vi "Insert.vi"(8 "error in (no error)":errorcluster, 9 "Item":refnum<class>, 10 "Index":i32, 11 "ListImp in":refnum<class "ListImp.lvclass">) -> (0 "error out":errorcluster, 3 "ListImp out":refnum<class "ListImp.lvclass">)   [LabVIEW 2013, in "LapDog.Collections.v1.Lists.lvlib" / "ListImp.lvclass"]
doc: "Inserts an item into the list at the location specified by Index, increasing the index of all items after the specified index by 1. If Index = -1 or Index = Count, the item is added to the end of the list. If Index < -1 or Index > Count, error 510201 is returned."
uses:
  ListImp.lvclass
  ListImp.lvclass/ListImp.ctl
  LapDog.Collections.Common/LapDog.Collections.v1.Common.lvlib
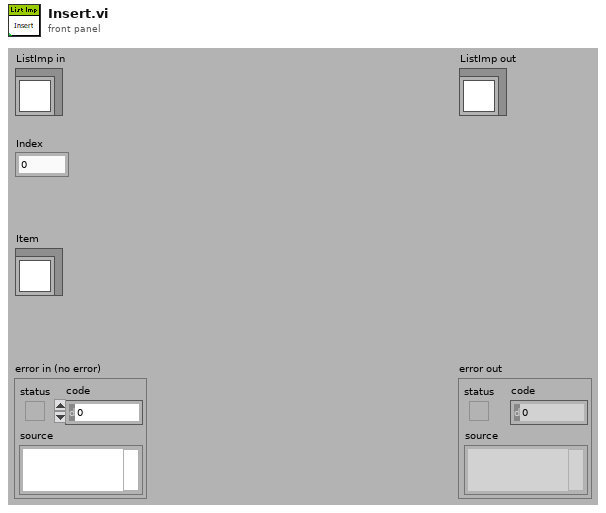
[diagram p1: front panel]
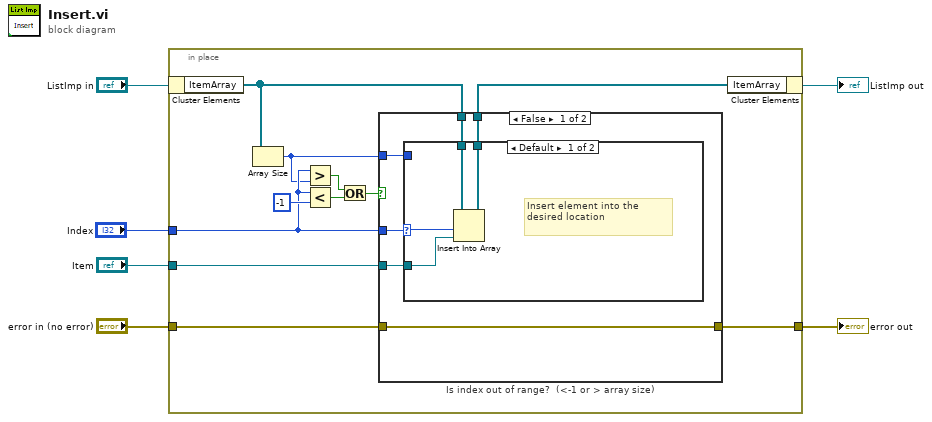
[diagram p0: block diagram]
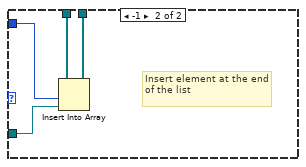
[diagram p2: hidden frame]
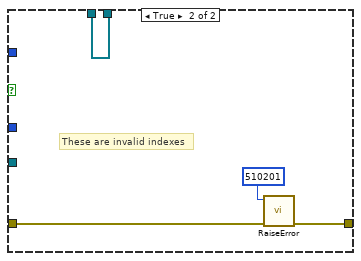
[diagram p3: hidden frame]
diagram:
  n1 = in-place {
    in-place-border: "Item" -> [w8]
    in-place-border: "Index" -> [w11]
    in-place-border: "error in (no error)" -> [w13]
    in-place-border: [w12] -> w3
    n2 = in-place-cluster #1("ListImp in") -> ("ItemArray"=w10:refnum<class>[])
    n3 = Array Size(array=w10) -> (size(s)=w7:i32)
    n4 = Greater?(x=w11, y=w7) -> (0:w15:bool)
    n5 = Less?(x=w11, y=-1) -> (x < y?=w16:bool)
    n6 = Or(x=w15, y=w16) -> (x .or. y?=w14:bool)
    n7 = case "Is index out of range?  (<-1 or > array size)" shown="False" w14 {
      tunnel: w13 -> [w23 w34]
      tunnel: [w23 w33] -> w12
      tunnel: w11 -> [w22 _]
      tunnel: w10 -> [w21 w32]
      tunnel: [w20 w32] -> w9
      tunnel: w8 -> [w19 _]
      tunnel: w7 -> [w18 _]
      frame False {
        n8 = case shown="Default" w22 {
          selector: w22 -> [w27 _]
          tunnel: w21 -> [w26 w31]
          tunnel: [w25 w28] -> w20
          tunnel: w19 -> [w24 w29]
          tunnel: w18 -> [_ w30]
          frame Default {
            # "Insert element into the desired location"
            n9 = Insert Into Array(array=w26, index=w27, new element=w24) -> (w25:refnum<class>[])
          }
          frame -1 {
            # "Insert element at the end of the list"
            n10 = Insert Into Array(array=w31, index=w30, new element=w29) -> (w28:refnum<class>[])
          }
        }
      }
      frame True {
        # "These are invalid indexes"
        n11 = call "RaiseError.vi"("error in (no error)"=w34, "Error Code"=510201) -> ("error out"=w33:errorcluster)  [unwired: 9 in]
      }
    }
    n12 = in-place-cluster #1("ItemArray"=w9) -> (→"ListImp out":refnum<class "ListImp.lvclass">)
  }
  "error out" <- w3
